vi "labview+arduino+leapmotion.vi"() -> ()   [LabVIEW 2015]
uses:
  <vilib>/MakerHub/LINX/Public/Peripherals/Digital/Digital Write N Chans.vi
  <vilib>/MakerHub/LINX/LMH-LINX.lvlib
  <vilib>/MakerHub/Leap/LMH-Leap.lvlib
panel:
  out "number of fingers":i32[](array[numeric])
  in  "stop":bool
  in  "Serial Port":refnum<visa-resource-name>="N/A"
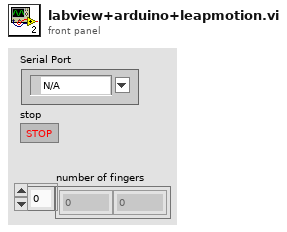
[diagram p1: front panel]
types:
  T1 = typedef "LMH-Leap.lvlib/Leap Handle.ctl" = cluster{"LeapCSharp":refnum<k24>}
  T2 = typedef "LMH-LINX.lvlib/LINX Ref.ctl" = cluster{"Platform":T3, "Interface":T4, "LINX Device Config":T5}
  T3 = typedef "LMH-LINX.lvlib/Platform.ctl" = enum16{"LINX", "myRIO"}
  T4 = typedef "LMH-LINX.lvlib/Interface.ctl" = enum16{"Serial", "TCP"}
  T5 = typedef "LMH-LINX.lvlib/Device.lvlib/LINX Device Config.ctl" = cluster{"Interface":T4, "COM Port":refnum<visa-resource-name>, "TCP Configuration":T6, "Device Family":u8, "Device ID":u8, "Device Name":string, "TCP Ref":refnum<k5>, "Channels":T7}
  T6 = typedef "LMH-LINX.lvlib/Device.lvlib/TCP Config.ctl" = cluster{"IP Address":string, "Port":u16}
  T7 = typedef "LMH-LINX.lvlib/Channels.ctl" = cluster{"DI":u8[], "DO":u8[], "AI":u8[], "AO":u8[], "PWM":u8[], "QE":u8[], "UART":u8[], "I2C 2":u8[], "SPI":u8[], "CAN":u8[], "Servo":u8[], "AI Ref (V)":dbl, "AO Ref (V)":dbl, "AO Resolution (Bits)":u8}
  T8 = typedef "LMH-Leap.lvlib/Frame.ctl" = cluster{"ID":i64, "Timestamp":i64, "Current FPS":dbl, "Key Tap Gestures":T9[], "Circle Gestures":T14[], "Screen Tap Gestures":T15[], "Swipe Gestures":T16[], "Hands":T17[]}
  T9 = typedef "LMH-Leap.lvlib/Gesture Key Tap.ctl" = cluster{"Common":T10, "Direction":T13, "Position":T13, "Progress":dbl}
  T10 = typedef "LMH-Leap.lvlib/Gesture Common.ctl" = cluster{"ID":dbl, "Duration (S)":dbl, "Gesture Type":T11, "Gesture State":T12}
  T11 = typedef "LMH-Leap.lvlib/Gesture Type.ctl" = enum16{"Invalid", "Swipe", "Circle", "Screen Tap", "Key Tap"}
  T12 = typedef "LMH-Leap.lvlib/Gesture State.ctl" = enum16{"Invalid", "Start", "Update", "Stop"}
  T13 = typedef "LMH-Leap.lvlib/Vector.ctl" = cluster{"Pitch":sgl, "Yaw":sgl, "Roll":sgl, "Magnitude":sgl, "XYZ":sgl[]}
  T14 = typedef "LMH-Leap.lvlib/Gesture Circle.ctl" = cluster{"Common":T10, "Center":T13, "Normal":T13, "Progress":dbl, "Radius":dbl}
  T15 = typedef "LMH-Leap.lvlib/Gesture Screen Tap.ctl" = cluster{"Common":T10, "Direction":T13, "Position":T13, "Progress":dbl}
  T16 = typedef "LMH-Leap.lvlib/Gesture Swipe.ctl" = cluster{"Common":T10, "Direction":T13, "Position":T13, "Start Position":T13, "Speed":dbl}
  T17 = typedef "LMH-Leap.lvlib/Hand.ctl" = cluster{"Palm Normal":T13, "Palm Position":T13, "Palm Velocity":T13, "Direction":T13, "Palm Position (Stabilized)":T13, "Sphere Center":T13, "Pointables":T18[], "ID":i32, "Time Visible":sgl, "Sphere Radius":sgl}
  T18 = typedef "LMH-Leap.lvlib/Pointable.ctl" = cluster{"Type":T19, "Touch Zone":T20, "ID":i32, "Length":dbl, "Width":dbl, "Time Visible":dbl, "Touch Distance":dbl, "Direction":T13, "Tip Position":T13, "Tip Velocity":T13, "Tip Position (Stabilized)":T13}
  T19 = typedef "LMH-Leap.lvlib/Pointable Type.ctl" = enum16{"Finger", "Tool"}
  T20 = typedef "LMH-Leap.lvlib/Pointable Zone.ctl" = enum16{"None", "Hovering", "Touching"}
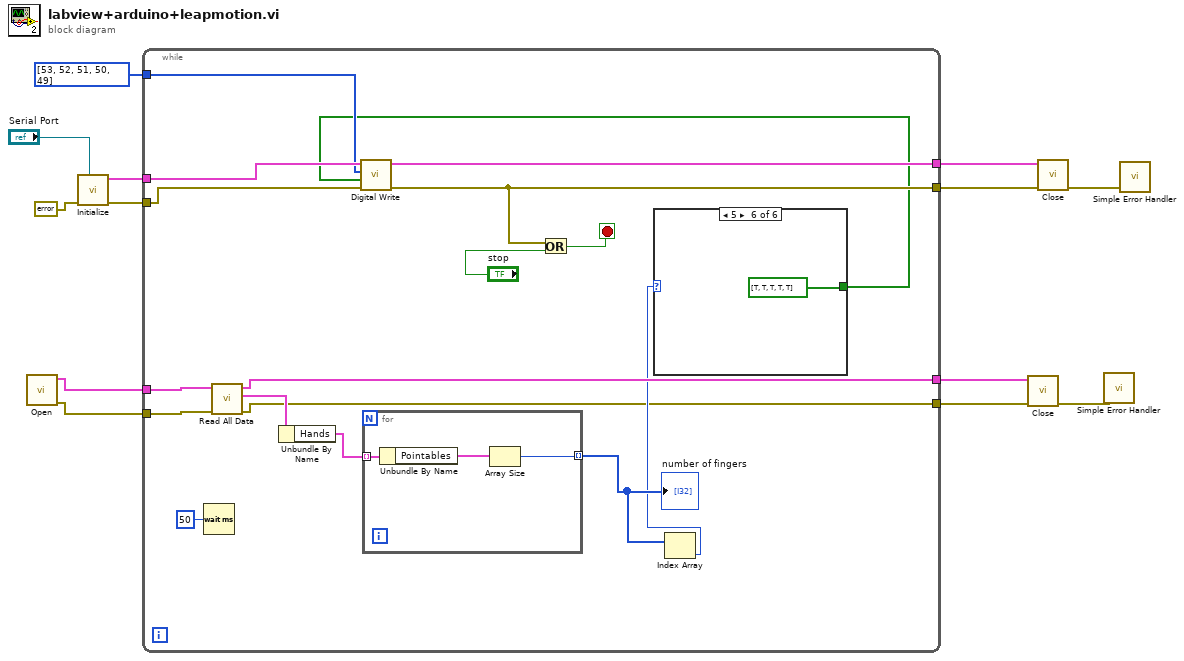
[diagram p0: block diagram]
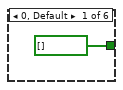
[diagram p2: hidden frame]
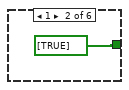
[diagram p3: hidden frame]
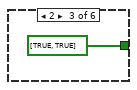
[diagram p4: hidden frame]
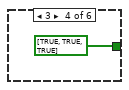
[diagram p5: hidden frame]
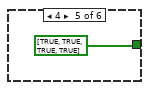
[diagram p6: hidden frame]
diagram:
  n1 = call <vilib>:"Open.vi"() -> ("Error Out"=w4:errorcluster, "Leap Handle"=w5:T1)  [unwired: 10 in]
  n2 = call <vilib>:"Initialize.vi"("Serial Port"="Serial Port", "Error In"=errorcluster {"status"=FALSE, "code"=0, "source"=""}) -> ("Error Out"=w9:errorcluster, "LINX Ref"=w10:T2)  [unwired: 7 in, 1 out]
  n3 = while {
    tunnel: w10 -> [w30]
    tunnel: w9 -> [w16]
    tunnel: [w29] -> w8
    tunnel: [w27] -> w7
    tunnel: w5 -> [w24]
    tunnel: w4 -> [w23]
    tunnel: [w22] -> w3
    tunnel: u8[] [53, 52, 51, 50, 49] ("DO Channels") -> [w17]
    tunnel: [w15] -> w1
    stop <- w28 stop-if-true
    n4 = Wait (ms)(milliseconds to wait=u32 50) -> ()  [unwired: 1 out]
    n5 = call <vilib>:"Read All Data.vi"("Error In"=w23, "Leap Handle"=w24) -> ("Error Out"=w15:errorcluster, "Frame"=w21:T8, "Leap Handle"=w22:T1)  [unwired: 6 in, 1 out]
    n6 = Unbundle By Name(w21) -> ("Hands"=w20:T17[])
    n7 = for {
      tunnel: w20 -> [w39] mode=indexing
      tunnel: [w37] -> w19 mode=indexing
      n8 = Unbundle By Name(w39) -> ("Pointables"=w38:T18[])
      n9 = Array Size(array=w38) -> (size(s)=w37:i32)
    }
    "number of fingers" <- w19
    n10 = Index Array(array=w19) -> (element=w18:i32)  [unwired: 1 in]
    n11 = case shown="5" w18 {
      tunnel: [bool[] [] bool[] [TRUE] bool[] [TRUE, TRUE] bool[] [TRUE, TRUE, TRUE] bool[] [TRUE, TRUE, TRUE, TRUE] bool[] [TRUE, TRUE, TRUE, TRUE, TRUE]] -> w14
      frame 0, Default {
      }
      frame 1 {
      }
      frame 2 {
      }
      frame 3 {
      }
      frame 4 {
      }
      frame 5 {
      }
    }
    n12 = call-poly <vilib>:"Digital Write.vi"("Error In"=w16, "Values"=w14, "DO Channels"=w17, "LINX Resource"=w30) -> ("Error Out"=w27:errorcluster, "LINX Resource"=w29:T2)  [unwired: 6 in]
    n13 = Or(x=w27, y="stop") -> (x .or. y?=w28:bool)
  }
  n14 = call <vilib>:"Close.vi"("Error In"=w1, "Leap Handle"=w3) -> ("Error Out"=w6:errorcluster)  [unwired: 9 in]
  n15 = call <vilib>:"Close.vi"("Error In"=w7, "LINX Resource"=w8) -> ("Error Out"=w11:errorcluster)  [unwired: 8 in, 1 out]
  n16 = call <vilib>:"Simple Error Handler.vi"("error in (no error)"=w6) -> ()  [unwired: 4 in, 5 out]
  n17 = call <vilib>:"Simple Error Handler.vi"("error in (no error)"=w11) -> ()  [unwired: 4 in, 5 out]
